vi "Constructor.vi"(10 "Beverage":refnum<class "Beverage.lvclass">, 11 "Soy in":refnum<class "Soy.lvclass">) -> (3 "Soy out":refnum<class "Soy.lvclass">)   [LabVIEW 2011, in "Soy.lvclass"]
uses:
  Soy.lvclass
  Beverage/Beverage.lvclass
  Soy.lvclass/Soy.ctl
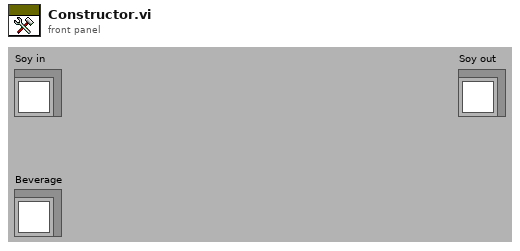
[diagram p1: front panel]
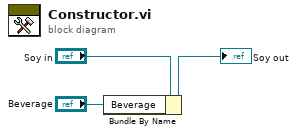
[diagram p0: block diagram]
diagram:
  n1 = Bundle By Name(cluster="Soy in", "Beverage"="Beverage") -> (→"Soy out":refnum<class "Soy.lvclass">)
